vi "HL7 Handle.vi"() -> ()   [LabVIEW 2016, in "main.lvlib"]
uses:
  main.lvlib
  HL7/HL7/HL7.lvclass
  C:/Program Files (x86)/National Instruments/LabVIEW 2016/vi.lib/ActorFramework/Actor/Actor.lvclass
  <vilib>/ActorFramework/Message Enqueuer/Message Enqueuer.lvclass/Message Enqueuer.ctl
  <vilib>/ActorFramework/Message Enqueuer/Enqueue.vi
  C:/Program Files (x86)/National Instruments/LabVIEW 2016/vi.lib/ActorFramework/Message/Message.lvclass
  <vilib>/ActorFramework/Stop Msg/Stop Msg.lvclass
  <vilib>/ActorFramework/Message Priority Queue/Priority Enqueue.vi
  EXO2/EXO2.lvlib
  <vilib>/ActorFramework/Actor/Actor.lvclass
panel:
  in  "open":bool
  in  "停止":bool
  in  "EXO message":T1
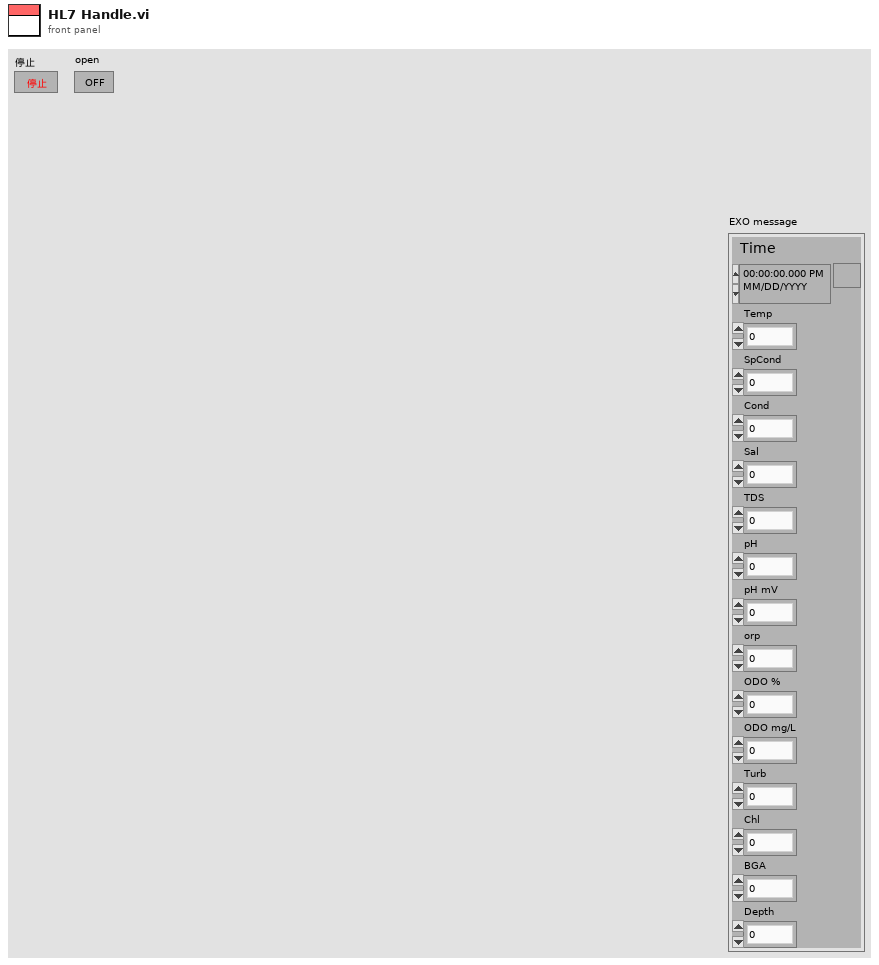
[diagram p1: front panel]
types:
  T1 = cluster{"Time":timestamp, "Temp":dbl, "SpCond":dbl, "Cond":dbl, "Sal":dbl, "TDS":dbl, "pH":dbl, "pH mV":dbl, "orp":dbl, "ODO %":dbl, "ODO mg/L":dbl, "Turb":dbl, "Chl":dbl, "BGA":dbl, "Depth":dbl}
  T2 = typedef "EXO2.lvlib/控件 1.ctl" = enum16{"open", "poll", "close", "run", "twipeb", "stop", "shutdown"}
  T3 = cluster{"Time":timestamp, "Temp":dbl, "SpCond":dbl, "Cond":dbl, "Sal":dbl, "TDS":dbl, "pH":dbl, "pH mV":dbl, "orp":dbl, "ODO %":dbl, "ODO mg/L":dbl, "Turb":dbl, "Chl":dbl, "BGA":dbl, "Depth":dbl}[]
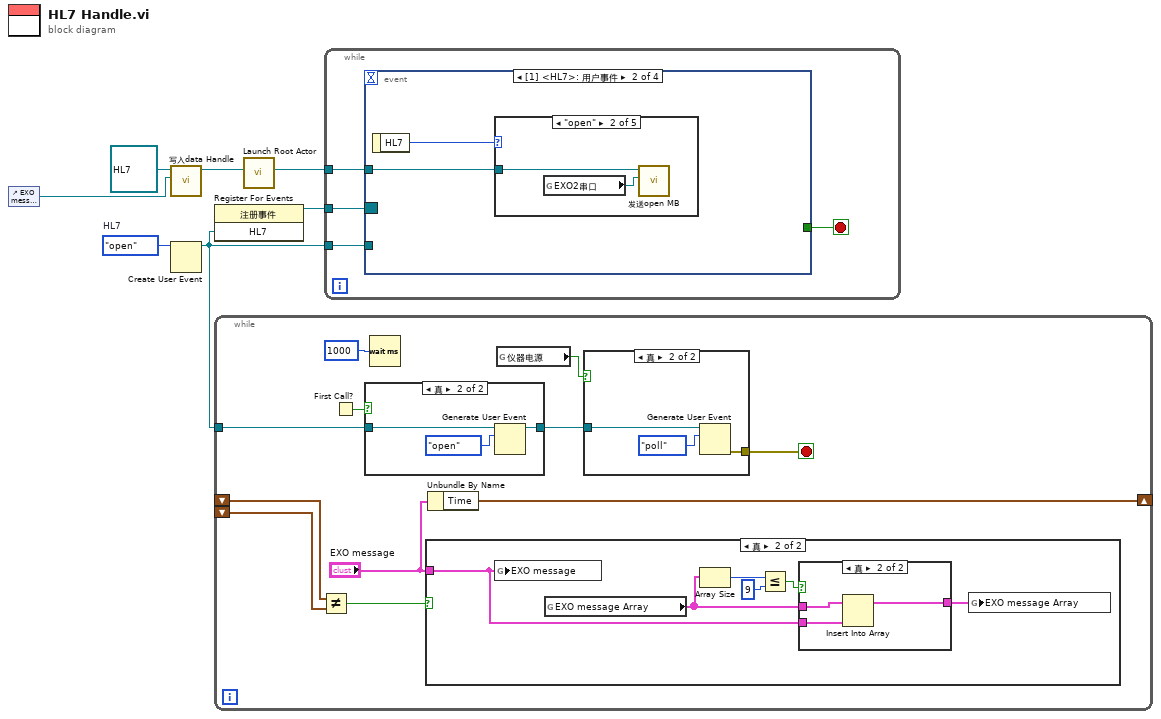
[diagram p0: block diagram]
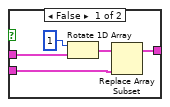
[diagram p5: hidden frame]
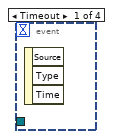
[diagram p6: hidden frame]
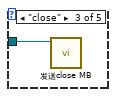
[diagram p8: hidden frame]
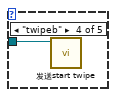
[diagram p9: hidden frame]
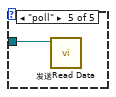
[diagram p10: hidden frame]
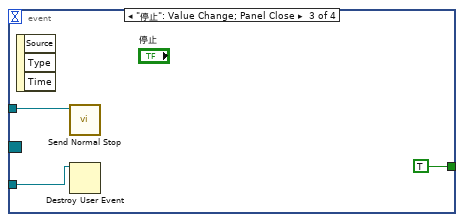
[diagram p11: hidden frame]
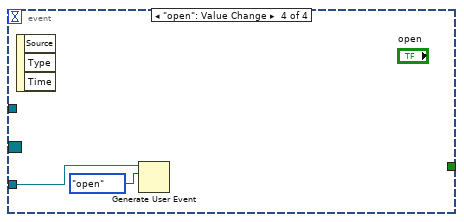
[diagram p12: hidden frame]
diagram:
  w4 = 控件_1."open"  # HL7
  n1 = control-ref of="EXO message"() -> (w6:refnum<vi>)
  n2 = call-dynamic "写入data Handle.vi"("data Handle"=w6, "HL7输入"=refnum<class "HL7.lvclass"> refnum ("HL7.lvlib:HL7.lvclass")) -> ("HL7输出"=w7:refnum<class "HL7.lvclass">)  [unwired: 8 in, 1 out]
  n3 = Create User Event(user event datatype=w4) -> (user event=w1:refnum<user-event>)  [unwired: 1 in, 1 out]
  n4 = register-events(w1) -> (reference out=w3:refnum<event-registration>)  [unwired: 2 in, 1 out]
  n5 = while {
    tunnel: w1 -> [w13]
    shift-right: [w9] -> _
    shift-left: _ -> [w14]
    shift-left: _ -> [w16]
    stop <- w18 stop-if-true
    n6 = Not Equal?(x=w14, y=w16) -> (x != y?=w15:bool)
    n7 = First Call?() -> (First Call?: T/F=w11:bool)
    n8 = case shown="真" w11 {
      tunnel: w13 -> [w22 w24]
      tunnel: [w22 w23] -> w12
      frame False {
      }
      frame True {
        n9 = Generate User Event(user event=w24, event data cluster=控件_1."open" ("事件数据")) -> (user event out=w23:refnum<user-event>)  [unwired: 2 in, 1 out]
      }
    }
    n10 = Wait (ms)(milliseconds to wait=u32 1000 ("等待时间（毫秒）")) -> ()  [unwired: 1 out]
    n11 = case shown="真" w15 {
      tunnel: "EXO message" -> [_ w26]
      frame False {
      }
      frame True {
        n12 = global write "EXO2全局变量.vi" "EXO message"(w26) -> ()
        n13 = global read "EXO2全局变量.vi" "EXO message Array"() -> (w28:T3)
        n14 = Array Size(array=w28) -> (size(s)=w29:i32)
        n15 = Less Or Equal?(x=w29, y=9) -> (x <= y?=w31:bool)
        n16 = case shown="真" w31 {
          tunnel: w26 -> [w33 w39]
          tunnel: [w32 w38] -> w27
          tunnel: w28 -> [w36 w37]
          frame False {
            n17 = Rotate 1D Array(1:w36, 2:1 ("n")) -> (0:w34:T3)
            n18 = Replace Array Subset(array=w34, new element=w33) -> (w32:T3)  [unwired: 1 in]
          }
          frame True {
            n19 = Insert Into Array(array=w37, new element=w39) -> (w38:T3)  [unwired: 1 in]
          }
        }
        n20 = global write "EXO2全局变量.vi" "EXO message Array"(w27) -> ()
      }
    }
    n21 = Unbundle By Name("EXO message") -> ("Time"=w9:timestamp)
    n22 = global read "全局非断电保持变量.vi" "仪器电源"() -> (w8:bool)
    n23 = case shown="真" w8 {
      tunnel: [_ w20] -> w18
      tunnel: w12 -> [_ w19]
      frame False {
      }
      frame True {
        n24 = Generate User Event(user event=w19, event data cluster=控件_1."poll" ("事件数据")) -> (error out=w20:errorcluster)  [unwired: 2 in, 1 out]
      }
    }
  }
  n25 = call <vilib>:"Launch Root Actor.vi"("Actor"=w7) -> ("Actor's Enqueuer"=w2:refnum<class "Message Enqueuer.lvclass">)  [unwired: 9 in, 1 out]
  n26 = while {
    tunnel: w2 -> [w42]
    tunnel: w3 -> [w41]
    tunnel: w1 -> [w40]
    stop <- w43 stop-if-true
    n27 = event shown="[1] <HL7>: 用户事件" {
      selector: w41 -> [_ _ _ _]
      dyn-events: _ -> [_ _ _ _]
      timeout: _ -> [_ _ _ _]
      tunnel: [_ _ TRUE _] -> w43
      tunnel: w42 -> [_ w44 w52 _]
      tunnel: w40 -> [_ _ w51 w55]
      event Timeout {
        n28 = event-data() -> ()  [unwired: 1 in, 3 out]
      }
      event User Event {
        n29 = event-data() -> ("HL7"=w45:T2)  [unwired: 1 in]
        n30 = case shown="\"open\"" w45 {
          tunnel: w44 -> [_ w47 w48 w49 w50]
          frame Default {
          }
          frame "open" {
            n31 = global read "EXO2全局变量.vi" "EXO2串口"() -> (w46:refnum<visa-resource-name>)
            n32 = call "发送open MB.vi"("VISA Resource"=w46, "Message Enqueuer"=w47) -> ()  [unwired: 8 in, 2 out]
          }
          frame "close" {
            n33 = call "发送close MB.vi"("Message Enqueuer"=w48) -> ()  [unwired: 9 in, 2 out]
          }
          frame "twipeb" {
            n34 = call "发送start twipe.vi"("Message Enqueuer"=w49) -> ()  [unwired: 9 in, 2 out]
          }
          frame "poll" {
            n35 = call "发送Read Data.vi"("Message Enqueuer"=w50) -> ()  [unwired: 9 in, 2 out]
          }
        }
      }
      event "停止": Value Change; Panel Close {
        n36 = event-data() -> ()  [unwired: 1 in, 3 out]
        n37 = call <vilib>:"Send Normal Stop.vi"("Message Enqueuer"=w52) -> ()  [unwired: 10 in, 1 out]
        n38 = Destroy User Event(user event=w51) -> ()  [unwired: 1 in, 1 out]
      }
      event "open": Value Change {
        n39 = event-data() -> ()  [unwired: 1 in, 3 out]
        n40 = Generate User Event(user event=w55, event data cluster=控件_1."open" ("事件数据")) -> ()  [unwired: 2 in, 2 out]
      }
    }
  }
